vi "Check Kings Status.vi"(0 "1D Board":T2[](array[typedef]), 5 "DT Team":i32, 11 "error in (no error)":errorcluster) -> (3 "Swap to Kill Opp. King?":bool, 4 "Opp. King in Danger?":bool, 6 "DT King in Danger?":bool, 8 "Opp. King Danger Cell":i32, 10 "DT King Danger Cell":i32, 15 "error out":errorcluster)   [LabVIEW 2014, in "Dragon Tamers.lvlib"]
uses:
  Dragon Tamers.lvlib
  Typedefs/Board Cell.ctl
  Typedefs/Cell Occupancy.ctl
  Typedefs/Debug Board 2D String.ctl
panel:
  in  "Debug?":bool
  in  "Table Control":T1
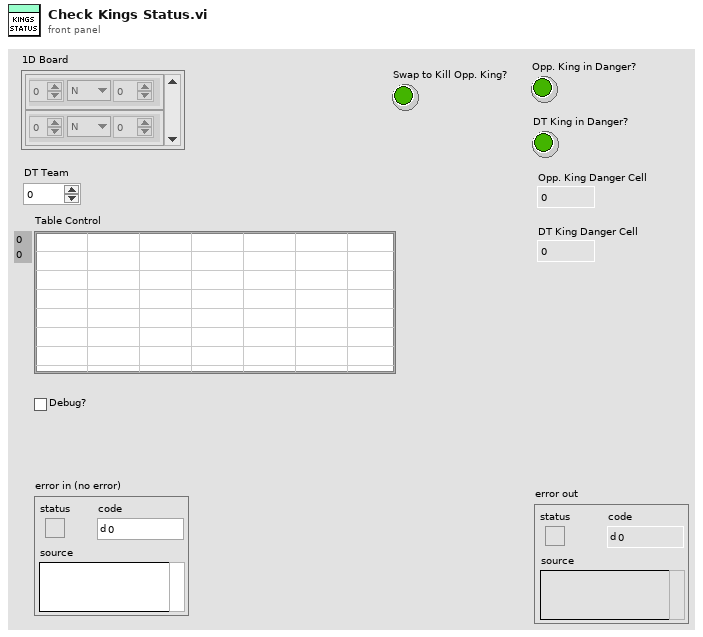
[diagram p1: front panel]
types:
  T1 = typedef "Dragon Tamers.lvlib/Debug Board 2D String.ctl" = string[][]
  T2 = typedef "Dragon Tamers.lvlib/Board Cell.ctl" = cluster{"Team":i32, "Occu.":T3, "Count":i32}
  T3 = typedef "Dragon Tamers.lvlib/Cell Occupancy.ctl" = enum16{"N", "C", "K"}
  T4 = typedef "Dragon Tamers.lvlib/Parsed Board.ctl" = cluster{"DT King":i32, "Opp King":i32, "Count":i32[], "Empty Cells":i32[], "DT Cells":i32[], "Opp Cells":i32[], "DT Team":i32, "Opp. Team":i32}
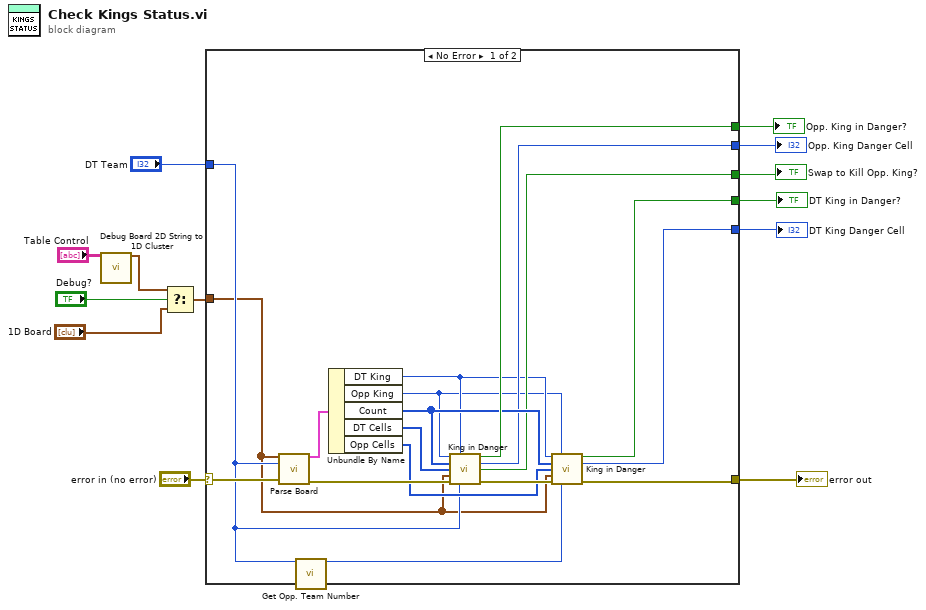
[diagram p0: block diagram]
diagram:
  n1 = call "Debug Board 2D String to 1D Cluster.vi"("Debug Board 2D String"="Table Control") -> ("1D Board"=w3:T2[])  [unwired: 14 in]
  n2 = Select(t=w3, s="Debug?", f="1D Board") -> (s? t:f=w1:T2[])
  n3 = case shown="No Error" "error in (no error)" {
    selector: "error in (no error)" -> [w31 w32]
    tunnel: [w24 w32] -> w12
    tunnel: "DT Team" -> [w16 _]
    tunnel: [w28 _] -> w10
    tunnel: [w25 _] -> w9
    tunnel: [w23 _] -> w8
    tunnel: [w22 _] -> w7
    tunnel: [w19 _] -> w6
    tunnel: w1 -> [w14 _]
    frame No Error {
      n4 = call "Parse Board.vi"("Board Array"=w14, "DT Team #"=w16, "error in (no error)"=w31) -> ("Parsed Board Info"=w30:T4, "error out"=w29:errorcluster)  [unwired: 11 in]
      n5 = call "Get Opp. Team Number.vi"("DT Team"=w16) -> ("Opp Team"=w15:i32)  [unwired: 14 in]
      n6 = Unbundle By Name(w30) -> ("DT King"=w18:i32, "Opp King"=w17:i32, "Count"=w26:i32[], "DT Cells"=w21:i32[], "Opp Cells"=w20:i32[])
      n7 = call "King in Danger.vi"("King Index"=w17, "Opp. King Index"=w18, "Count"=w26, "Opp Team Cells"=w21, "1D Board"=w14, "error in (no error)"=w29, "Team"=w16) -> ("King in Danger?"=w28:bool, "Cell Index"=w23:i32, "Swap to Kill?"=w19:bool, "error out"=w27:errorcluster)  [unwired: 5 in]
      n8 = call "King in Danger.vi"("King Index"=w18, "Opp. King Index"=w17, "Count"=w26, "Opp Team Cells"=w20, "1D Board"=w14, "error in (no error)"=w27, "Team"=w15) -> ("King in Danger?"=w25:bool, "Cell Index"=w22:i32, "error out"=w24:errorcluster)  [unwired: 5 in, 1 out]
    }
    frame Error {
    }
  }
  "error out" <- w12
  "Opp. King in Danger?" <- w10
  "DT King in Danger?" <- w9
  "Opp. King Danger Cell" <- w8
  "DT King Danger Cell" <- w7
  "Swap to Kill Opp. King?" <- w6
